vi "MTS_SaveColorImagePng.vi"(5 "Save .png":bool=TRUE, 6 "Tree Refnum":refnum<vi>, 7 ".pt3 File Name":path, 8 "error in":errorcluster, 9 "Colors":u32[](array[numeric]), 10 "Active":bool[](array[boolean]), 11 "Image":i32[][][](array[numeric])) -> (0 "error out":errorcluster)   [LabVIEW 2010]
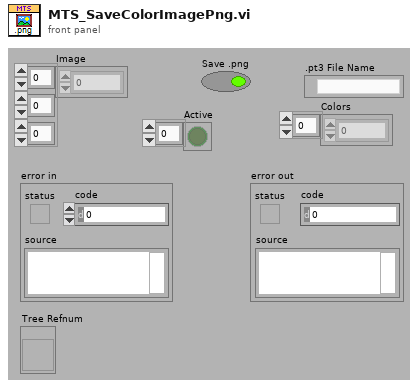
[diagram p1: front panel]
types:
  T1 = enum16{"unknown", "pt3 File", "png Image", "bmp Image"}
  T2 = enum16{"not a pt3 File", "Image File", "Point Measurement", "Auto Point"}
  T3 = typedef "Image Type" = u32
  T4 = typedef "IMAQ Image.ctl" = refnum<image>
  T5 = cluster{"File No":i32, "File Path":path, "Parent File":i32, "File Type":enum16{"unknown", "pt3 File", "png Image", "bmp Image"}, "Measurement Type":enum16{"not a pt3 File", "Image File", "Point Measurement", "Auto Point", "Line Scan", "Grid Scan"}, "Upper Left":cluster{"x-Position":dbl, "y-Position":dbl, "z-Position":dbl}, "Pixels":i32[], "Picture Size":dbl[], "Scan Axis":enum32{"x-y", "x-z", "y-z"}}
  T6 = cluster{"x-Position":dbl, "y-Position":dbl, "z-Position":dbl}
  T7 = cluster{"Picture Size":dbl[], "Pixels":i32[], "Upper Left":cluster{"x-Position":dbl, "y-Position":dbl, "z-Position":dbl}}
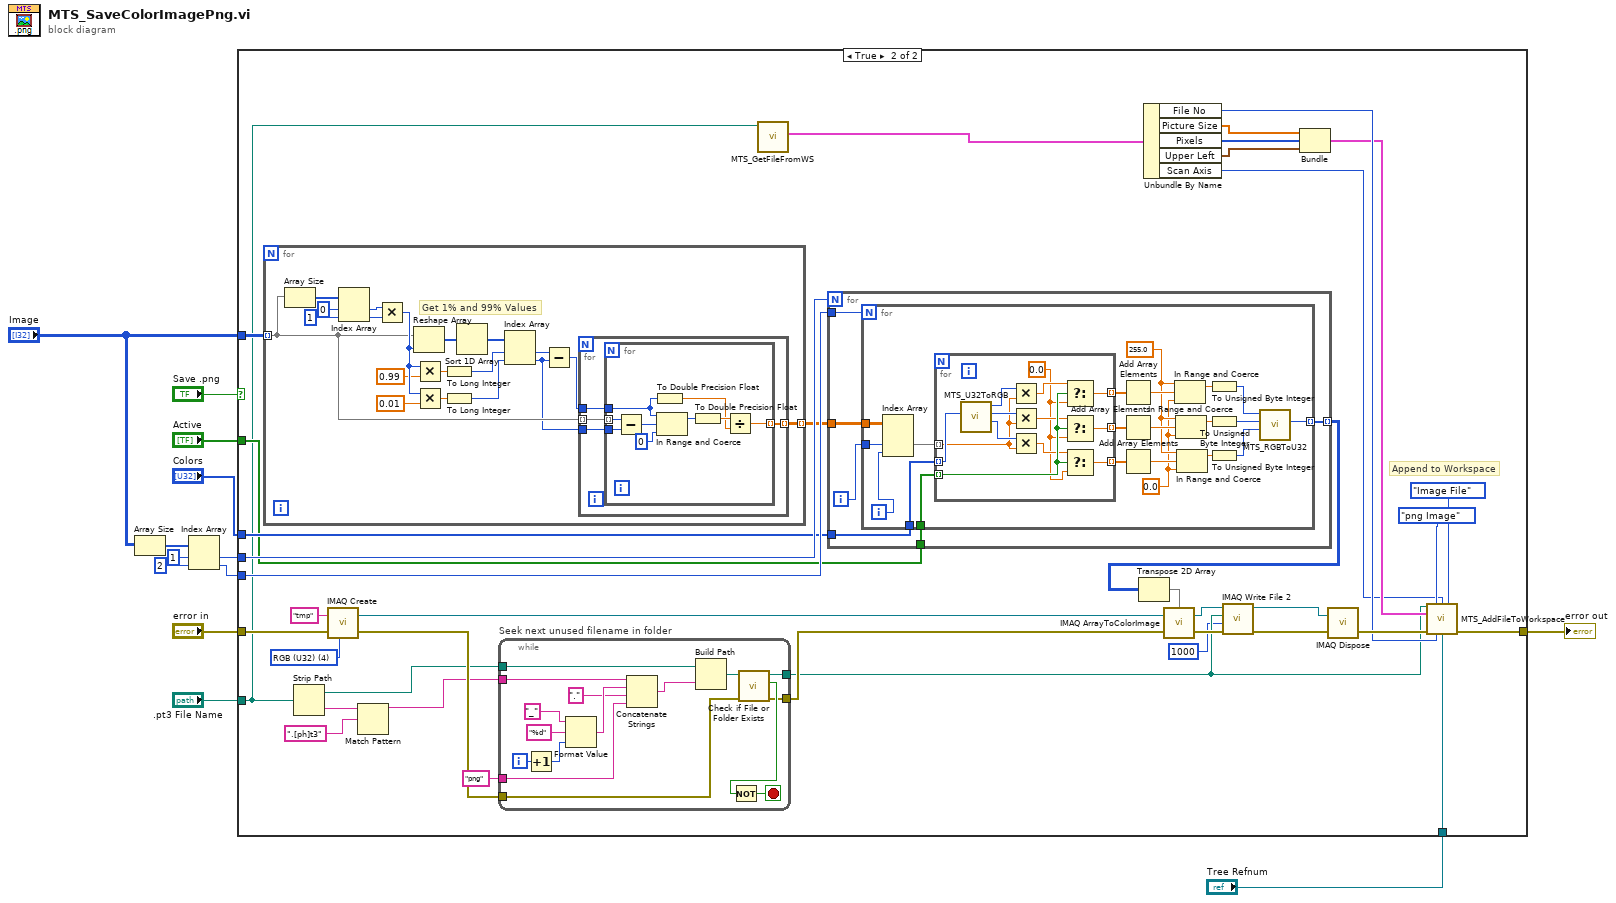
[diagram p0: block diagram]
diagram:
  n1 = Array Size(array="Image") -> (size(s)=w8:i32[])
  n2 = Index Array(array=w8, index #1=1 ("index"), index #2=2 ("index")) -> (element #1=w4:i32, element #2=w3:i32)
  n3 = case shown="True" "Save .png" {
    tunnel: "Image" -> [_ w49]
    tunnel: "error in" -> [w14 w52]
    tunnel: [w14 w35] -> w11
    tunnel: ".pt3 File Name" -> [_ w17]
    tunnel: "Tree Refnum" -> [_ w34]
    tunnel: w4 -> [_ w24]
    tunnel: w3 -> [_ w23]
    tunnel: "Colors" -> [_ w21]
    tunnel: "Active" -> [_ w20]
    frame False {
    }
    frame True {
      w50 = T3 4 items=["Grayscale (U8)", "Grayscale (I16)", "Grayscale (SGL)", "Complex (CSG)", "RGB (U32)", "HSL (U32)", "RGB (U64)", "Grayscale (U16)"] ("Image Type")
      # "Append to Workspace"
      n4 = for {
        tunnel: w49 -> [w97] mode=indexing
        tunnel: [w93] -> w22 mode=indexing
        # "Get 1% and 99% Values"
        n5 = Array Size(array=w97) -> (size(s)=w111:i32[])
        n6 = Index Array(array=w111, index #1=0 ("index"), index #2=1 ("index")) -> (element #1=w108:i32, element #2=w107:i32)
        n7 = Multiply(x=w108, y=w107) -> (x*y=w104:i32)
        n8 = Reshape Array(w97, w104) -> (w106:i32[])
        n9 = Multiply(x=w104, y=0.99) -> (x*y=w101:dbl)
        n10 = Multiply(x=w104, y=0.01) -> (x*y=w100:dbl)
        n11 = To Long Integer(number=w101) -> (32bit integer=w98:i32)
        n12 = To Long Integer(number=w100) -> (32bit integer=w99:i32)
        n13 = Sort 1D Array(array=w106) -> (sorted array=w105:i32[])
        n14 = Index Array(array=w105, index #1=w98, index #2=w99) -> (element #1=w96:i32, element #2=w95:i32)
        n15 = Subtract(x=w96, y=w95) -> (x-y=w94:i32)
        n16 = for {
          tunnel: w97 -> [w115] mode=indexing
          tunnel: w95 -> [w114]
          tunnel: w94 -> [w113]
          tunnel: [w112] -> w93 mode=indexing
          n17 = for {
            tunnel: w115 -> [w124] mode=indexing
            tunnel: w114 -> [w123]
            tunnel: w113 -> [w119]
            tunnel: [w116] -> w112 mode=indexing
            n18 = Subtract(x=w124, y=w123) -> (x-y=w122:i32)
            n19 = To Double Precision Float(number=w119) -> (double precision float=w117:dbl)
            n20 = In Range and Coerce(upper limit=w119, x=w122, lower limit=0) -> (coerced(x)=w120:i32)  [unwired: 1 out]
            n21 = To Double Precision Float(number=w120) -> (double precision float=w118:dbl)
            n22 = Divide(x=w118, y=w117) -> (x/y=w116:dbl)
          }
        }
      }
      n23 = Strip Path(path=w17) -> (stripped path=w39:path, name=w43:string)
      n24 = call "IMAQ Create"("Image Name"="tmp", "Image Type"=w50, "error in (no error)"=w52) -> ("New Image"=w48:T4, "error out"=w41:errorcluster)  [unwired: 1 in, 1 out]
      n25 = Match Pattern(string=w43, regular expression=".[ph]t3") -> (before substring=w38:string)  [unwired: 4 out]
      n26 = while "Seek next unused filename in folder" {
        tunnel: w39 -> [w140]
        tunnel: [w135] -> w27
        tunnel: w41 -> [w134]
        tunnel: [w133] -> w40
        tunnel: w38 -> [w128]
        tunnel: "png" ("File Type") -> [w125]
        i -> [w130]
        stop <- w137 stop-if-true
        n27 = Increment(x=w130) -> (x+1=w129:i32)
        n28 = Format Value(string ("")="_", format string="%d", value (0)=w129) -> (output string=w131:string)
        n29 = Concatenate Strings(w128, w131, "." ("string"), w125) -> (w139:string)
        n30 = Build Path(base path=w140, name or relative path=w139) -> (appended path=w138:path)
        n31 = call <vilib>:"Check if File or Folder Exists.vi"("error in (no error)"=w134, "path"=w138) -> ("error out"=w133:errorcluster, "file or folder exists?"=w136:bool, "dup path"=w135:path)  [unwired: 7 out]
        n32 = Not(x=w136) -> (.not. x?=w137:bool)
      }
      n33 = call "MTS_GetFileFromWS.vi"(".pt3 File Name"=w17) -> ("File Header"=w16:T5)  [unwired: 9 in, 1 out]
      n34 = for {
        N: w24 -> [_]
        tunnel: w23 -> [w58]
        tunnel: w22 -> [w57]
        tunnel: w21 -> [w55]
        tunnel: w20 -> [w54]
        tunnel: [w53] -> w18 mode=indexing
        i -> [w56]
        n35 = for {
          N: w58 -> [_]
          tunnel: w57 -> [w79]
          tunnel: w56 -> [w78]
          tunnel: w55 -> [w76]
          tunnel: w54 -> [w74]
          tunnel: [w59] -> w53 mode=indexing
          i -> [w77]
          w66 = 0.0 ("lower limit")
          w67 = 255.0 ("upper limit")
          n36 = Index Array(array=w79, index (dim 1)=w78, index (dim 2)=w77) -> (element=w75:dbl[])  [unwired: 1 in]
          n37 = for {
            tunnel: w76 -> [w92] mode=indexing
            tunnel: w75 -> [w88] mode=indexing
            tunnel: w74 -> [w86] mode=indexing
            tunnel: [w82] -> w73 mode=indexing
            tunnel: [w81] -> w72 mode=indexing
            tunnel: [w80] -> w71 mode=indexing
            w83 = 0.0 ("f")
            n38 = call "MTS_U32ToRGB.vi"("Color"=w92) -> ("Blue"=w89:u8, "Green"=w90:u8, "Red"=w91:u8)  [unwired: 8 out]
            n39 = Multiply(x=w91, y=w88) -> (x*y=w87:dbl)
            n40 = Multiply(x=w90, y=w88) -> (x*y=w85:dbl)
            n41 = Multiply(x=w89, y=w88) -> (x*y=w84:dbl)
            n42 = Select(t=w87, s=w86, f=w83) -> (s? t:f=w82:dbl)
            n43 = Select(t=w85, s=w86, f=w83) -> (s? t:f=w81:dbl)
            n44 = Select(t=w84, s=w86, f=w83) -> (s? t:f=w80:dbl)
          }
          n45 = Add Array Elements(numeric array=w73) -> (sum=w70:dbl)
          n46 = Add Array Elements(numeric array=w72) -> (sum=w69:dbl)
          n47 = Add Array Elements(numeric array=w71) -> (sum=w68:dbl)
          n48 = In Range and Coerce(upper limit=w67, x=w70, lower limit=w66) -> (coerced(x)=w65:dbl)  [unwired: 1 out]
          n49 = In Range and Coerce(upper limit=w67, x=w69, lower limit=w66) -> (coerced(x)=w64:dbl)  [unwired: 1 out]
          n50 = In Range and Coerce(upper limit=w67, x=w68, lower limit=w66) -> (coerced(x)=w63:dbl)  [unwired: 1 out]
          n51 = To Unsigned Byte Integer(number=w65) -> (unsigned 8bit integer=w62:u8)
          n52 = To Unsigned Byte Integer(number=w64) -> (unsigned 8bit integer=w61:u8)
          n53 = To Unsigned Byte Integer(number=w63) -> (unsigned 8bit integer=w60:u8)
          n54 = call "MTS_RGBToU32.vi"("Blue"=w60, "Green"=w61, "Red"=w62) -> ("Color"=w59:u32)  [unwired: 8 out]
        }
      }
      n55 = Transpose 2D Array(2D array=w18) -> (transposed array=w19:u32[][])
      n56 = Unbundle By Name(w16) -> ("File No"=w29:i32, "Picture Size"=w32:dbl[], "Pixels"=w31:i32[], "Upper Left"=w30:T6, "Scan Axis"=w15:enum32{"x-y", "x-z", "y-z"})
      n57 = call "IMAQ ArrayToColorImage"("Image Pixels (U32)"=w19, "Image"=w48, "error in (no error)"=w40) -> ("Image Out"=w45:T4, "error out"=w47:errorcluster)  [unwired: 1 in, 1 out]
      n58 = call-poly "IMAQ Write File 2"("error in (no error)"=w47, "Image Quality"=u32 1000, "File Path"=w27, "Image"=w45) -> ("error out"=w46:errorcluster, "Image Out (duplicate)"=w44:T4)  [unwired: 2 in, 4 out]
      n59 = Bundle("Picture Size"=w32, "Pixels"=w31, "Upper Left"=w30) -> (w28:T7)  [unwired: 1 out]
      n60 = call "IMAQ Dispose"("Image"=w44, "error in (no error)"=w46) -> ("error out"=w36:errorcluster)  [unwired: 1 in, 3 out]
      n61 = call "MTS_AddFileToWorkspace.vi"("File Name"=w27, "File Type"=T1."png Image", "Scan Axis"=w15, "Measurement Type"=T2."Image File", "File Info"=w28, "error in (no error)"=w36, "Parent"=w29, "Tree Refnum"=w34) -> ("error out"=w35:errorcluster)  [unwired: 7 out]
    }
  }
  "error out" <- w11
